vi "Tegam4040 -- GetDriverVersion.vi"(8 "error in (no error)":errorcluster) -> (0 "error out":errorcluster, 3 "Driver Version":string)   [LabVIEW 2010]
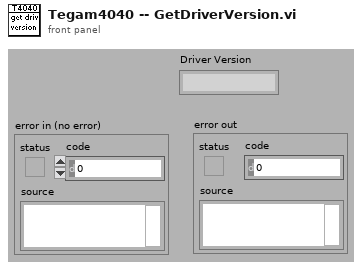
[diagram p1: front panel]
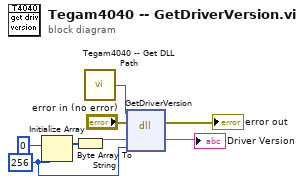
[diagram p0: block diagram]
diagram:
  w7 = 256 ("dimension size")
  n1 = Initialize Array(u8 0, w7) -> (w6:u8[])
  n2 = Byte Array To String(unsigned byte array=w6) -> (string=w5:string)
  n3 = call "Tegam4040 -- Get DLL Path.vi"() -> ("DLL Path"=w1:path)  [unwired: 8 in]
  n4 = dll-call lib="G:/My Documents/T4040/Tegam4040CDriver/release/Tegam4040CDriver.dll" fn="GetDriverVersion"(path in=w1, error in="error in (no error)", "stringBuf"=w5, "bufLength"=w7) -> (error out=→"error out":errorcluster, "stringBuf"=→"Driver Version":string)  [unwired: 3 in, 1 out]
